vi "1.vi"   [LabVIEW 2018]
uses:
  <vilib>/Analysis/polynomials.llb/Polynomial Roots (DBL).vi
  <vilib>/Analysis/NI_AALPro.lvlib
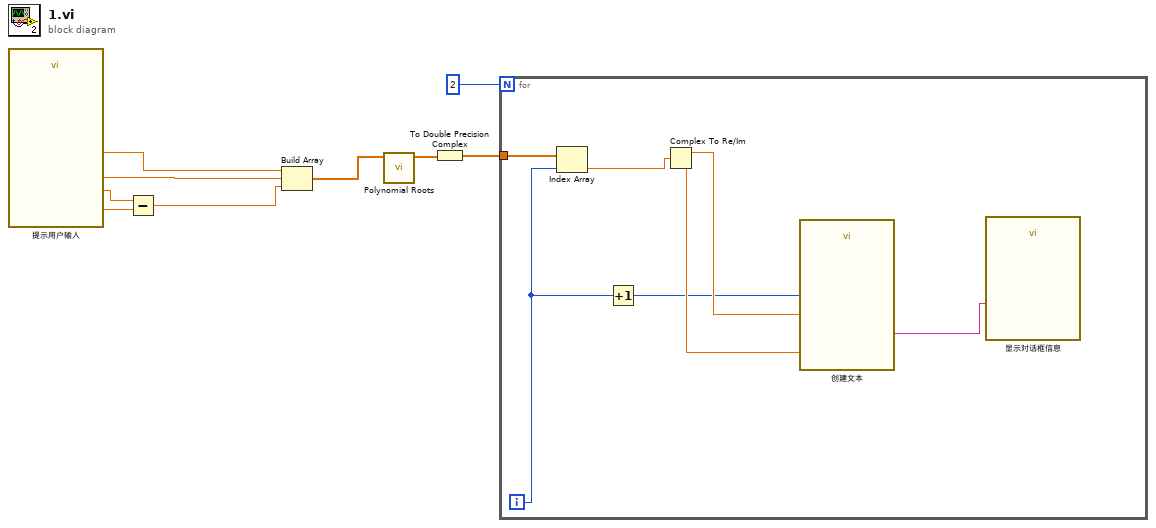
[diagram p0: block diagram]
diagram:
  n1 = call "提示用户输入"() -> ("D"=w5:dbl, "C"=w6:dbl, "B"=w8:dbl, "A"=w9:dbl)  [unwired: 14 in, 2 out]
  n2 = Subtract(x=w6, y=w5) -> (x-y=w4:dbl)
  n3 = Build Array(w9, w8, w4) -> (w7:dbl[])
  n4 = call-poly <vilib>:"Polynomial Roots.vi"("P(x)"=w7) -> ("Roots"=w3:cdb[])  [unwired: 9 in, 1 out]
  n5 = To Double Precision Complex(1:w3) -> (0:w2:cdb[])
  n6 = for {
    N: 2 -> [_]
    tunnel: w2 -> [w16]
    i -> [w11]
    n7 = Index Array(array=w16, index=w11) -> (element=w15:cdb)
    n8 = Increment(x=w11) -> (x+1=w10:i32)
    n9 = Complex To Re/Im(x + iy=w15) -> (x=w13:dbl, y=w12:dbl)
    n10 = call "创建文本"("c"=w10, "a"=w13, "b"=w12) -> ("Result"=w14:string)  [unwired: 11 in, 1 out]
    n11 = call "显示对话框信息"("Message"=w14) -> ()  [unwired: 9 in, 2 out]
  }
